vi "LibXML_SaveXML.vi"(8 "error in":errorcluster, 9 "file path (dialog if empty)":path, 11 "doc":u32) -> (0 "error out":errorcluster, 2 "bytes written":i32, 3 "doc copy out":u32)   [LabVIEW 2019, in "Tools.lvlib" / "LibXML.lvlib"]
doc: "Backs up old file and saves the document to file. The Document will not be closed and the references are still valid"
uses:
  LibXML.lvlib
  dll/libxml2.dll
panel:
  # "This software is FREE licensed under the GNU Lesser General Public License"
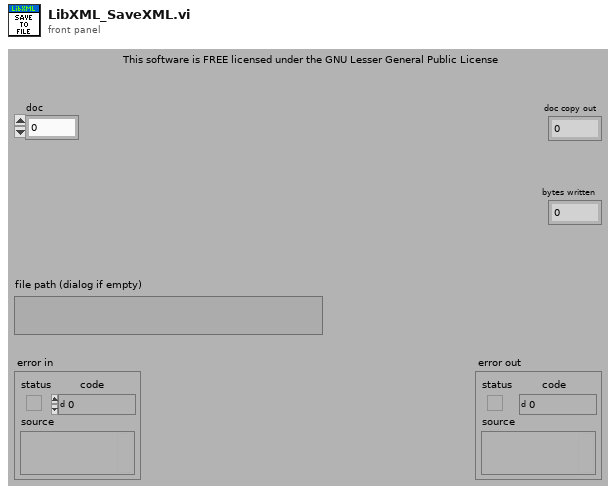
[diagram p1: front panel]
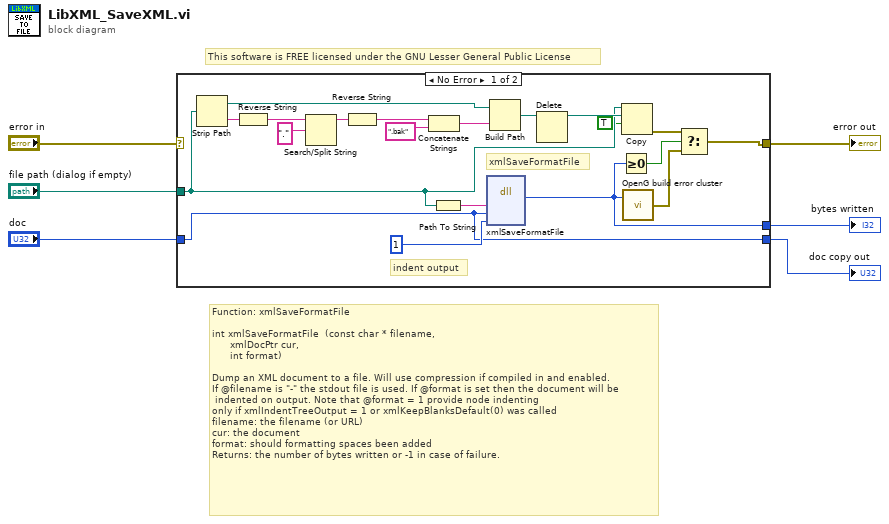
[diagram p0: block diagram]
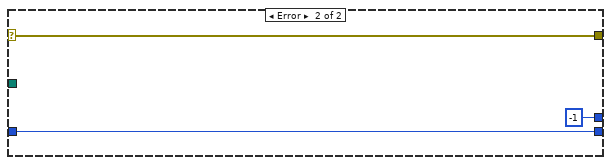
[diagram p2: hidden frame]
diagram:
  # "Function: xmlSaveFormatFile\n\nint\txmlSaveFormatFile\t\t(const char * filename, \n\t\t\t\t\t xmlDocPtr cur, \n\t\t\t\t\t int format)\n\nDump an XML document to a file. Will use compression if compiled in and enabled. \nIf @filename is \"-\" the stdout file is used. If @format is set then the document will be\n indented on output. Note that @format = 1 provide node indenting \nonly if xmlIndentTreeOutput = 1 or xmlKeepBlanksDefault(0) was called\nfilename:\tthe filename (or URL)\ncur:\tthe document\nformat:\tshould formatting spaces been added\nReturns:\tthe number of bytes written or -1 in case of failure."
  # "This software is FREE licensed under the GNU Lesser General Public License"
  n1 = case shown="No Error" "error in" {
    selector: "error in" -> [_ w29]
    tunnel: [w11 w29] -> w6
    tunnel: "doc" -> [w15 w28]
    tunnel: [w15 w28] -> w3
    tunnel: [w10 -1 ("return type")] -> w2
    tunnel: "file path (dialog if empty)" -> [w9 _]
    frame No Error {
      # "indent output"
      # "xmlSaveFormatFile"
      n2 = Strip Path(path=w9) -> (stripped path=w22:path, name=w26:string)
      n3 = Reverse String(1:w26) -> (0:w19:string)
      n4 = Search/Split String(string=w19, search string/char (-)=".") -> (substring before match=w24:string)  [unwired: 1 in, 2 out]
      n5 = Reverse String(1:w24) -> (0:w18:string)
      n6 = Concatenate Strings(w18, ".bak") -> (w23:string)
      n7 = Path To String(path=w9) -> (string=w16:string)
      n8 = dll-call lib="C:/Projects/_Prywatne/MyCIT/Framework/Tools/XML/LibXML/dll/libxml2.dll" fn="xmlSaveFormatFile"("filename"=w16, "doc"=w15, "style"=1) -> ("return type"=w10:i32)  [unwired: 6 in, 2 out]
      n9 = Build Path(base path=w22, name or relative path=w23) -> (appended path=w21:path)
      n10 = Delete(path (use dialog)=w21) -> (deleted path=w20:path)  [unwired: 4 in, 2 out]
      n11 = Greater Or Equal To 0?(x=w10) -> (x >= 0?=w13:bool)
      n12 = Copy(9:TRUE ("overwrite (F)"), 10:w20, 11:w9) -> (0:w8:errorcluster)  [unwired: 2 in, 2 out]
      n13 = call "OpenG build error cluster.vi"("code"=w10) -> ("error out"=w12:errorcluster)  [unwired: 1 in]
      n14 = Select(t=w8, s=w13, f=w12) -> (s? t:f=w11:errorcluster)
    }
    frame Error {
    }
  }
  "error out" <- w6
  "doc copy out" <- w3
  "bytes written" <- w2
